vi "DoPaint.vi"(8 "error in (no error)":errorcluster, 11 "White in":refnum<class "White.lvclass">) -> (0 "error out":errorcluster, 3 "White out":refnum<class "White.lvclass">)   [LabVIEW 2014, in "White.lvclass"]
uses:
  White.lvclass
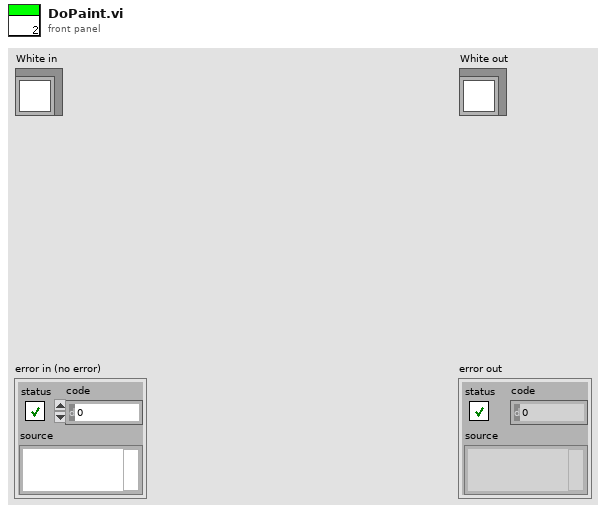
[diagram p1: front panel]
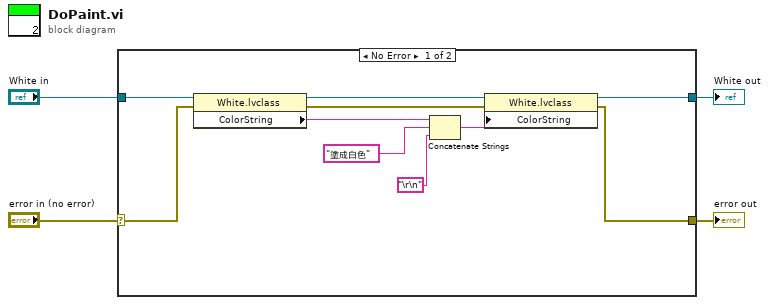
[diagram p0: block diagram]
diagram:
  n1 = case shown="No Error" "error in (no error)" {
    selector: "error in (no error)" -> [w14 w16]
    tunnel: [w11 w16] -> w4
    tunnel: [w9 w15] -> w3
    tunnel: "White in" -> [w12 w15]
    frame No Error {
      n2 = property class="White.lvclass"(reference=w12, error in=w14) -> (reference out=w10:refnum<class "White.lvclass">, error out=w13:errorcluster, "ColorString"=w8:string)
      n3 = Concatenate Strings(w8, "塗成白色" ("string"), "\r\n" ("string")) -> (w7:string)
      n4 = property class="White.lvclass"(reference=w10, error in=w13, "ColorString"=w7) -> (reference out=w9:refnum<class "White.lvclass">, error out=w11:errorcluster)
    }
    frame Error {
    }
  }
  "error out" <- w4
  "White out" <- w3
